vi "GetConfigDataSTD.vi"(0 "object in":refnum<class "AFG3022B_OJ.lvclass">, 5 "error in (no error)":errorcluster) -> (14 "object out":refnum<class "AFG3022B_OJ.lvclass">, 16 "Configdatastd":T1, 19 "error out":errorcluster)   [LabVIEW 2023, in "AFG3022B_OJ.lvclass"]
uses:
  AFG3022B_OJ.lvclass
  AFG3022B_OJ.lvclass/AFG3022B_OJ.ctl
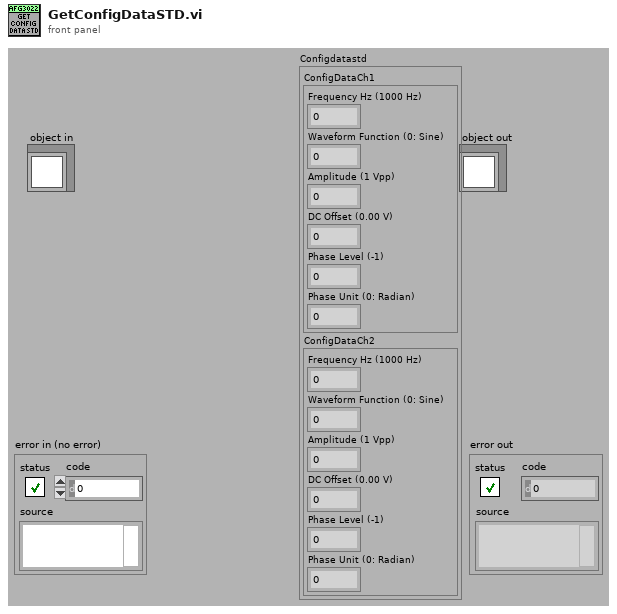
[diagram p1: front panel]
types:
  T1 = cluster{"ConfigDataCh1":cluster{"Frequency Hz (1000 Hz)":dbl, "Waveform Function (0: Sine)":u16, "Amplitude (1 Vpp)":dbl, "DC Offset (0.00 V)":dbl, "Phase Level (-1)":dbl, "Phase Unit (0: Radian)":u16}, "ConfigDataCh2":cluster{"Frequency Hz (1000 Hz)":dbl, "Waveform Function (0: Sine)":u16, "Amplitude (1 Vpp)":dbl, "DC Offset (0.00 V)":dbl, "Phase Level (-1)":dbl, "Phase Unit (0: Radian)":u16}}
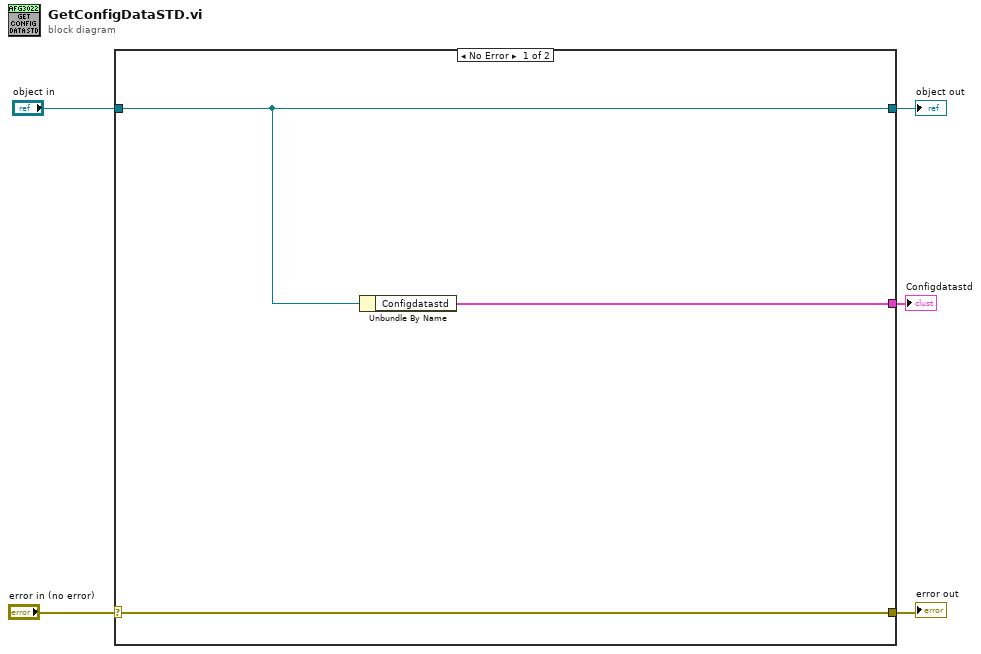
[diagram p0: block diagram]
diagram:
  n1 = case shown="No Error" "error in (no error)" {
    selector: "error in (no error)" -> [w7 w10]
    tunnel: [w7 w10] -> w4
    tunnel: [w6 w9] -> w2
    tunnel: "object in" -> [w6 w9]
    tunnel: [w8 _] -> w1
    frame No Error {
      n2 = Unbundle By Name(w6) -> ("Configdatastd"=w8:T1)
    }
    frame Error {
    }
  }
  "error out" <- w4
  "object out" <- w2
  "Configdatastd" <- w1
